vi "Asynchorous autofocus.vi"() -> ()   [LabVIEW 2014]
uses:
  autofocus-globals.vi
panel:
  in  "Delay (s)":dbl
  in  "Stop Program":bool
  in  "Run?":bool
  # "Press OK to run autofocusing. Make sure to press STOP to abort execution."
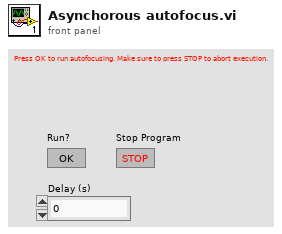
[diagram p1: front panel]
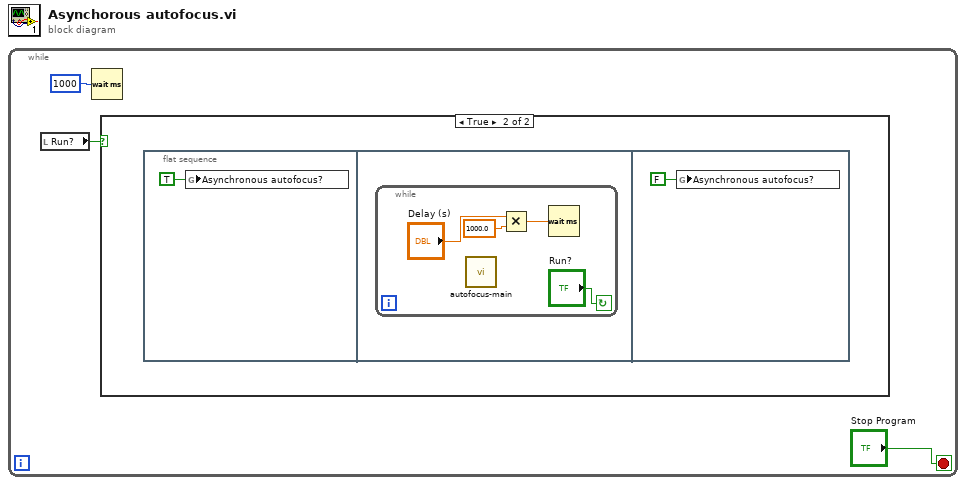
[diagram p0: block diagram]
diagram:
  n1 = while {
    stop <- "Stop Program" stop-if-true
    n2 = local read "Run?"() -> (w2:bool)
    n3 = Wait (ms)(milliseconds to wait=u32 1000) -> ()  [unwired: 1 out]
    n4 = case shown="True" w2 {
      frame False {
      }
      frame True {
        n5 = flat-sequence {
          frame #0 {
            n6 = global write "autofocus-globals.vi" "Asynchronous autofocus?"(TRUE ("Asynchronous autofocus?")) -> ()
          }
          frame #1 {
            n7 = while {
              stop <- "Run?" continue-if-true
              n8 = call "autofocus-main.vi"() -> ()  [unwired: 12 in]
              n9 = Multiply(x="Delay (s)", y=1000.0) -> (x*y=w7:dbl)
              n10 = Wait (ms)(milliseconds to wait=w7) -> ()  [unwired: 1 out]
            }
          }
          frame #2 {
            n11 = global write "autofocus-globals.vi" "Asynchronous autofocus?"(FALSE ("Asynchronous autofocus?")) -> ()
          }
        }
      }
    }
  }
